vi "Auton Sequence2.vi"(6 "speed":dbl=0.7, 8 "AI 7 Feedback (inches)":dbl, 9 "AI 7 PWM Input":dbl, 10 "AI 5 Setpoint Secondary":dbl, 11 "AI 5 PWM Input":dbl) -> (2 "AI 7 PWM Output":dbl, 3 "AI 5 PWM Output":dbl)   [LabVIEW 2011]
uses:
  Robot Global Data.vi
panel:
  out "AI 7 Previous":dbl
  in  "Forced Retraction":dbl
  in  "Rotation Sequence":dbl
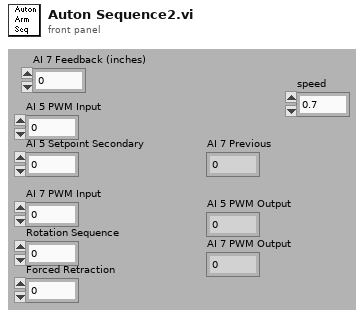
[diagram p1: front panel]
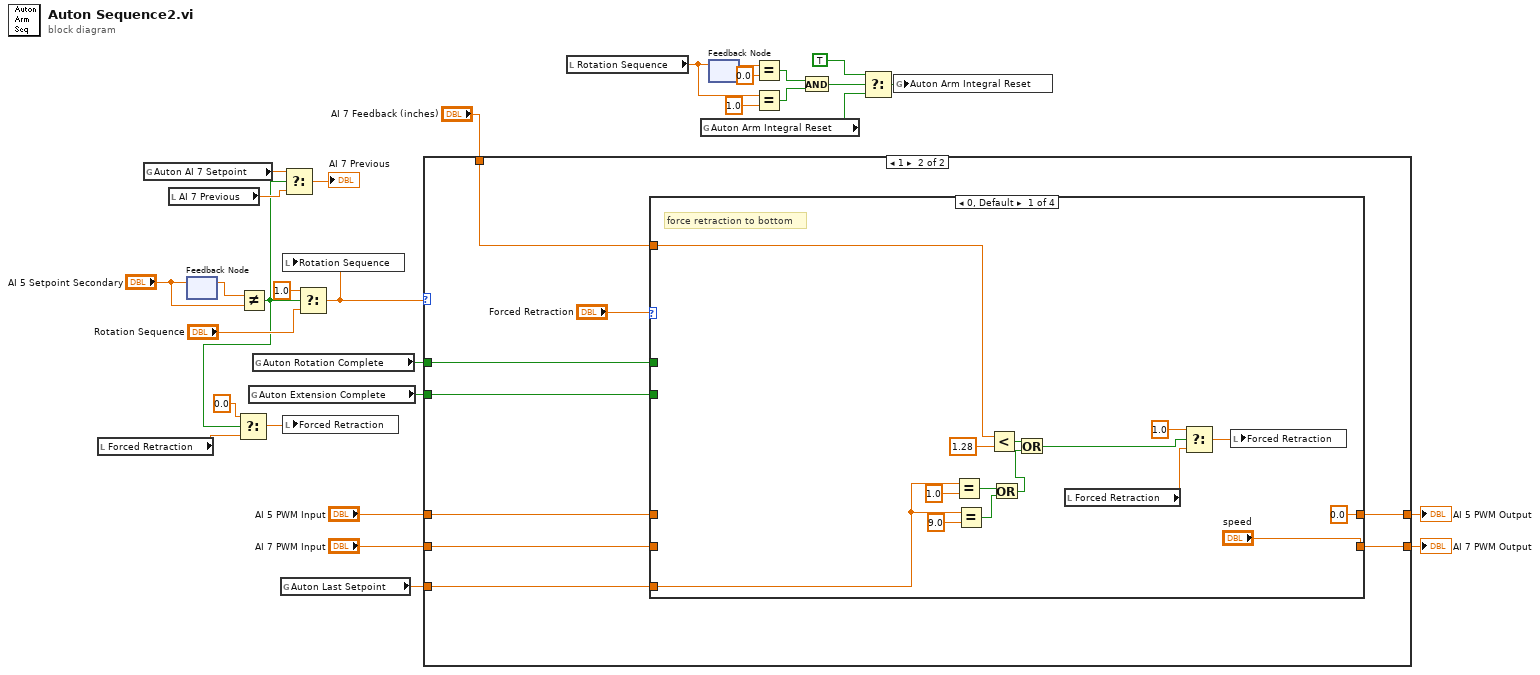
[diagram p0: block diagram]
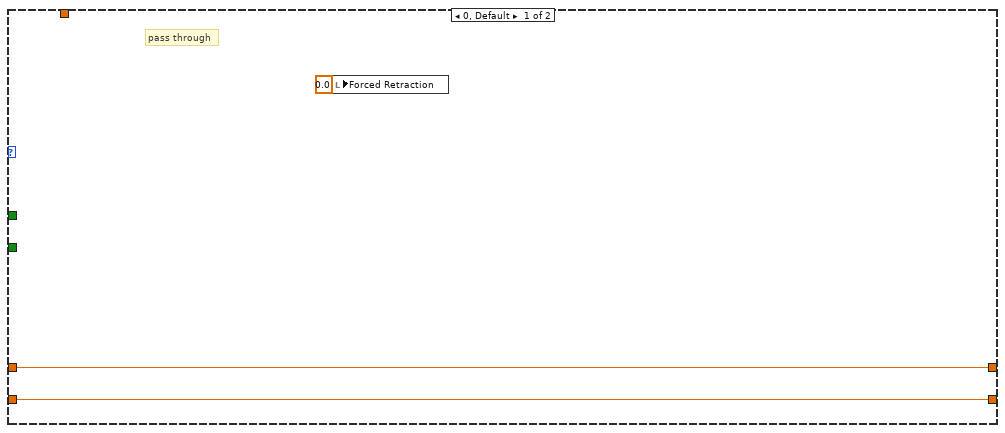
[diagram p2: hidden frame]
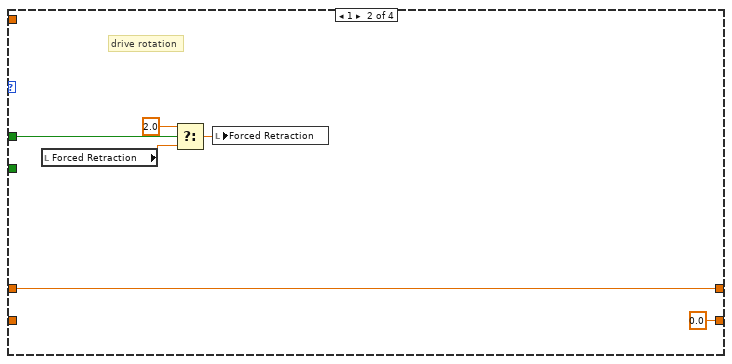
[diagram p3: hidden frame]
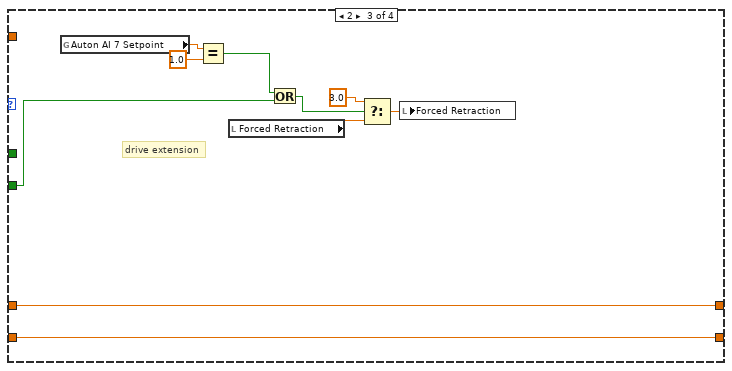
[diagram p4: hidden frame]
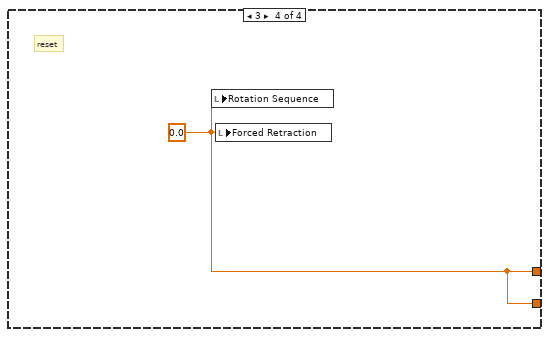
[diagram p5: hidden frame]
diagram:
  n1 = local read "Forced Retraction"() -> (w3:dbl)
  n2 = global read "Robot Global Data.vi" "Auton AI 7 Setpoint"() -> (w21:dbl)
  n3 = local read "AI 7 Previous"() -> (w19:dbl)
  n4 = feedback-in #1("AI 5 Setpoint Secondary") -> ()
  n5 = feedback #1() -> (w30:dbl)  [unwired: 1 out]
  n6 = Not Equal?(x=w30, y="AI 5 Setpoint Secondary") -> (x != y?=w5:bool)
  n7 = Select(t=0.0, s=w5, f=w3) -> (s? t:f=w2:dbl)
  n8 = global read "Robot Global Data.vi" "Auton Extension Complete"() -> (w7:bool)
  n9 = global read "Robot Global Data.vi" "Auton Rotation Complete"() -> (w18:bool)
  n10 = global read "Robot Global Data.vi" "Auton Last Setpoint"() -> (w1:dbl)
  n11 = local write "Forced Retraction"(w2) -> ()
  n12 = Select(t=w21, s=w5, f=w19) -> (s? t:f=→"AI 7 Previous":dbl)
  n13 = Select(t=1.0, s=w5, f="Rotation Sequence") -> (s? t:f=w22:dbl)
  n14 = local write "Rotation Sequence"(w22) -> ()
  n15 = case shown="1" w22 {
    tunnel: "AI 5 PWM Input" -> [w33 w38]
    tunnel: "AI 7 PWM Input" -> [w32 w42]
    tunnel: [w33 w39] -> w25
    tunnel: [w32 w41] -> w24
    tunnel: w18 -> [_ w37]
    tunnel: w7 -> [_ w36]
    tunnel: "AI 7 Feedback (inches)" -> [_ w35]
    tunnel: w1 -> [_ w34]
    frame 0, Default {
      # "pass through"
      n16 = local write "Forced Retraction"(0.0 ("Forced Retraction")) -> ()
    }
    frame 1 {
      n17 = case shown="0, Default" "Forced Retraction" {
        tunnel: w42 -> [_ _ w72 _]
        tunnel: ["speed" 0.0 ("AI 7 PWM Input") w72 w74] -> w41
        tunnel: [0.0 ("AI 5 PWM Input") w62 w73 w74] -> w39
        tunnel: w38 -> [_ w62 w73 _]
        tunnel: w37 -> [_ w61 _ _]
        tunnel: w36 -> [_ _ w67 _]
        tunnel: w35 -> [w55 _ _ _]
        tunnel: w34 -> [w44 _ _ _]
        frame 0, Default {
          # "force retraction to bottom"
          n18 = Equal?(x=w44, y=1.0) -> (x = y?=w47:bool)
          n19 = Equal?(x=w44, y=9.0) -> (x = y?=w46:bool)
          n20 = Less?(x=w55, y=1.28) -> (x < y?=w51:bool)
          n21 = Or(x=w47, y=w46) -> (x .or. y?=w45:bool)
          n22 = Or(x=w51, y=w45) -> (x .or. y?=w48:bool)
          n23 = local read "Forced Retraction"() -> (w53:dbl)
          n24 = Select(t=1.0, s=w48, f=w53) -> (s? t:f=w54:dbl)
          n25 = local write "Forced Retraction"(w54) -> ()
        }
        frame 1 {
          # "drive rotation"
          n26 = local read "Forced Retraction"() -> (w59:dbl)
          n27 = Select(t=2.0, s=w61, f=w59) -> (s? t:f=w58:dbl)
          n28 = local write "Forced Retraction"(w58) -> ()
        }
        frame 2 {
          # "drive extension"
          n29 = global read "Robot Global Data.vi" "Auton AI 7 Setpoint"() -> (w66:dbl)
          n30 = Equal?(x=w66, y=1.0 ("t")) -> (x = y?=w65:bool)
          n31 = local read "Forced Retraction"() -> (w70:dbl)
          n32 = Or(x=w65, y=w67) -> (x .or. y?=w68:bool)
          n33 = Select(t=3.0, s=w68, f=w70) -> (s? t:f=w69:dbl)
          n34 = local write "Forced Retraction"(w69) -> ()
        }
        frame 3 {
          w74 = 0.0 ("Forced Retraction")
          # "reset"
          n35 = local write "Rotation Sequence"(w74) -> ()
          n36 = local write "Forced Retraction"(w74) -> ()
        }
      }
    }
  }
  "AI 5 PWM Output" <- w25
  "AI 7 PWM Output" <- w24
  n37 = local read "Rotation Sequence"() -> (w15:dbl)
  n38 = global read "Robot Global Data.vi" "Auton Arm Integral Reset"() -> (w9:bool)
  n39 = feedback-in #2(w15) -> ()
  n40 = feedback #2() -> (w17:dbl)  [unwired: 1 out]
  n41 = Equal?(x=w17, y=0.0) -> (x = y?=w12:bool)
  n42 = Equal?(x=w15, y=1.0) -> (x = y?=w13:bool)
  n43 = And(x=w12, y=w13) -> (x .and. y?=w11:bool)
  n44 = Select(t=TRUE, s=w11, f=w9) -> (s? t:f=w8:bool)
  n45 = global write "Robot Global Data.vi" "Auton Arm Integral Reset"(w8) -> ()
